vi "Joystick_Operation.vi"(0 "System no.":i32=1 min=1 step=1, 1 "Joystick ID":u32, 2 "X axis":string="B", 3 "Y axis":string="E", 4 "No.of digits for MOV command":i16=2, 5 "error in":errorcluster, 6 "Resolution factor X":i32=150, 7 "Resolution factor Y":i32=150, 8 "Dead band X":i32=2, 9 "Dead band Y":i32=2, 10 "Use #24 for Stop?":bool=TRUE, 11 "Read from controller?":bool=TRUE caption="Read travel range\nfrom controller?", 12 "Maximum velocity values":T2={"Velocity1 X"=1.0, "Velocity2 X"=20.0, "Velocity1 Y"=0.5, "Velocity2 Y"=15.0} {"Velocity2 Y" format="%.6f"; "Velocity1 Y" format="%.6f"; "Velocity2 X" format="%.6f"; "Velocity1 X" format="%.6f"}, 13 "Travel range":T1={"Xmax"=10.0, "Xmin"=0.0, "Ymax"=5.0, "Ymin"=0.0} {"Ymin" format="%.6f"; "Ymax" format="%.6f"; "Xmin" format="%.6f"; "Xmax" format="%.6f"}, 14 "System no. 2":i32=1 min=1 step=1) -> (19 "error out":errorcluster)   [LabVIEW 2020]
doc: "This VI can be used to control two closed-loop axes (which can belong to one or two connected systems) with a 2-button, 2-axis joystick connected to the host computer. The absolute value of the joystick position is converted into velocity values for the two stages connected to the system being commanded. Two velocity levels for each axis can be specified, e.g. one for fast, rough positioning and one for slow, fine positioning. Joystick button 2 switches between these levels. The sign of the joystick position determines whether the move command issued contains the positive or negative travel limit (read automatically if Read travel range from controller? is TRUE) of the corresponding axis. When the joystick is \"in the middle position\", the velocity of the corresponding axis is set to zero. \nDead band * is the maximum size of the scaled joystick position value that does not result in any motion. \nResolution factor * determines the joystick resolution. \nNo. of digits is the number of digits after the decimal point in the position values that will be sent by the MOV command. \nIf joystick button 1 is pressed, a stop command (STP or #24, depending on Use 24 for stop) is sent to the controller. The diagram shows how to combine the driver and support VIs for these tasks. \n\nIf only one motion axis is to be controlled, Y Axis must be identical to X Axis, System no. 2 must be identical to System no. 1, and Y axis of joystick is to be used for control of the motion axis.\n\nIf required: Install the joystick driver and calibrate the joystick in the Windows control panel before running this VI.\n\nRun PI_GCS2_Configuration_setup.vi prior to running this VI."
uses:
  Low Level/General command.llb/Controller names.ctl
  Low Level/General command.llb/Global2 (Array).vi
panel:
  out "Current Vy":dbl(slide) scale=0.0..0.5 scale format="%.4f"
  out "Current Vx":dbl(slide) scale=0.0..1.0 scale format="%.4f"
  out "Position plot":cluster{dbl[], dbl[]}(graph)
  out "Current pos. Y":dbl format="%.2f"
  out "Current pos. X":dbl format="%.2f"
  out "Current Vy":dbl format="%.6f"
  out "Current Vx":dbl format="%.6f"
  out "Current Vy, max":dbl format="%.6f"
  out "Current Vx, max":dbl format="%.6f"
  in  "stop":bool
  out "JoyY":i32
  out "JoyX":i32
  out "JoyY scaled":i32
  out "JoyX scaled":i32
  # "Joystick operation sample program."
  # "Install joystick driver, calibrate joystick in the Windows control \tpanel and run \"Configuration_Setup.vi\" before running this VI. Use joystick button 1\nto stop motion of both axes and button2 to switch between two velocity levels. If only one motion axis is to be controlled, Y Axis must be identical\nto X Axis, System no. 2 must be identical to System no. 1, and Y axis of joystick is to be used for control of the motion axis.See VI and control/\nindicator information for details."
  # "For X axis:"
  # "For Y axis:"
  # "Joystick axes settings"
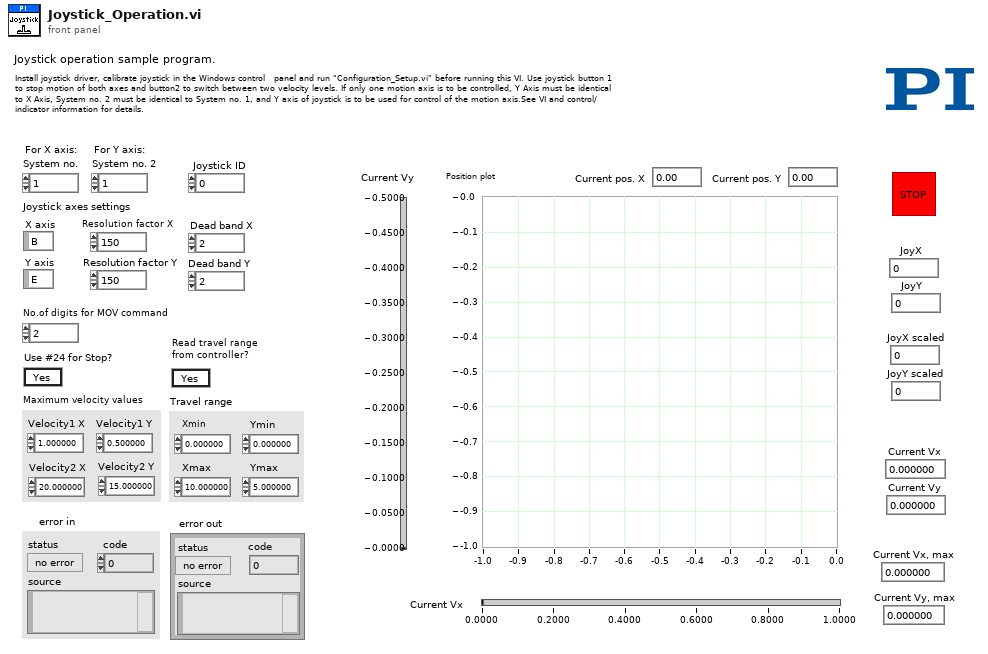
[diagram p1: front panel]
types:
  T1 = cluster{"Xmax":dbl, "Xmin":dbl, "Ymax":dbl, "Ymin":dbl}
  T2 = cluster{"Velocity1 X":dbl, "Velocity2 X":dbl, "Velocity1 Y":dbl, "Velocity2 Y":dbl}
  T3 = typedef "Controller names.ctl" = enum16{"None", "Analog", "C-702", "C-413", "C-414", "C-843", "C-843.PM", "C-844", "C-848", "C-865", "C-866", "C-867", "C-877", "C-880", "C-884", "C-885", "C-886", "C-887", "C-891", "E-135", "E-516", "E-517", "E-518", "E-709", "E-710", "E-712", "E-725", "E-727", "E-753", "E-754", "E-755", "E-761", "E-816", "E-861", "E-870", "E-871", "E-872", "E-873", "E-874", "F-206", "HydraPollux", "M-840", "M-850", "M-8X0", "Mercury", "Mercury_GCS", "PI_GCS2"}
  T4 = cluster{"Conn. axes":string[], "Controller name":T3}[]
  T5 = cluster{"Conn. axes":string[], "Controller name":T3}
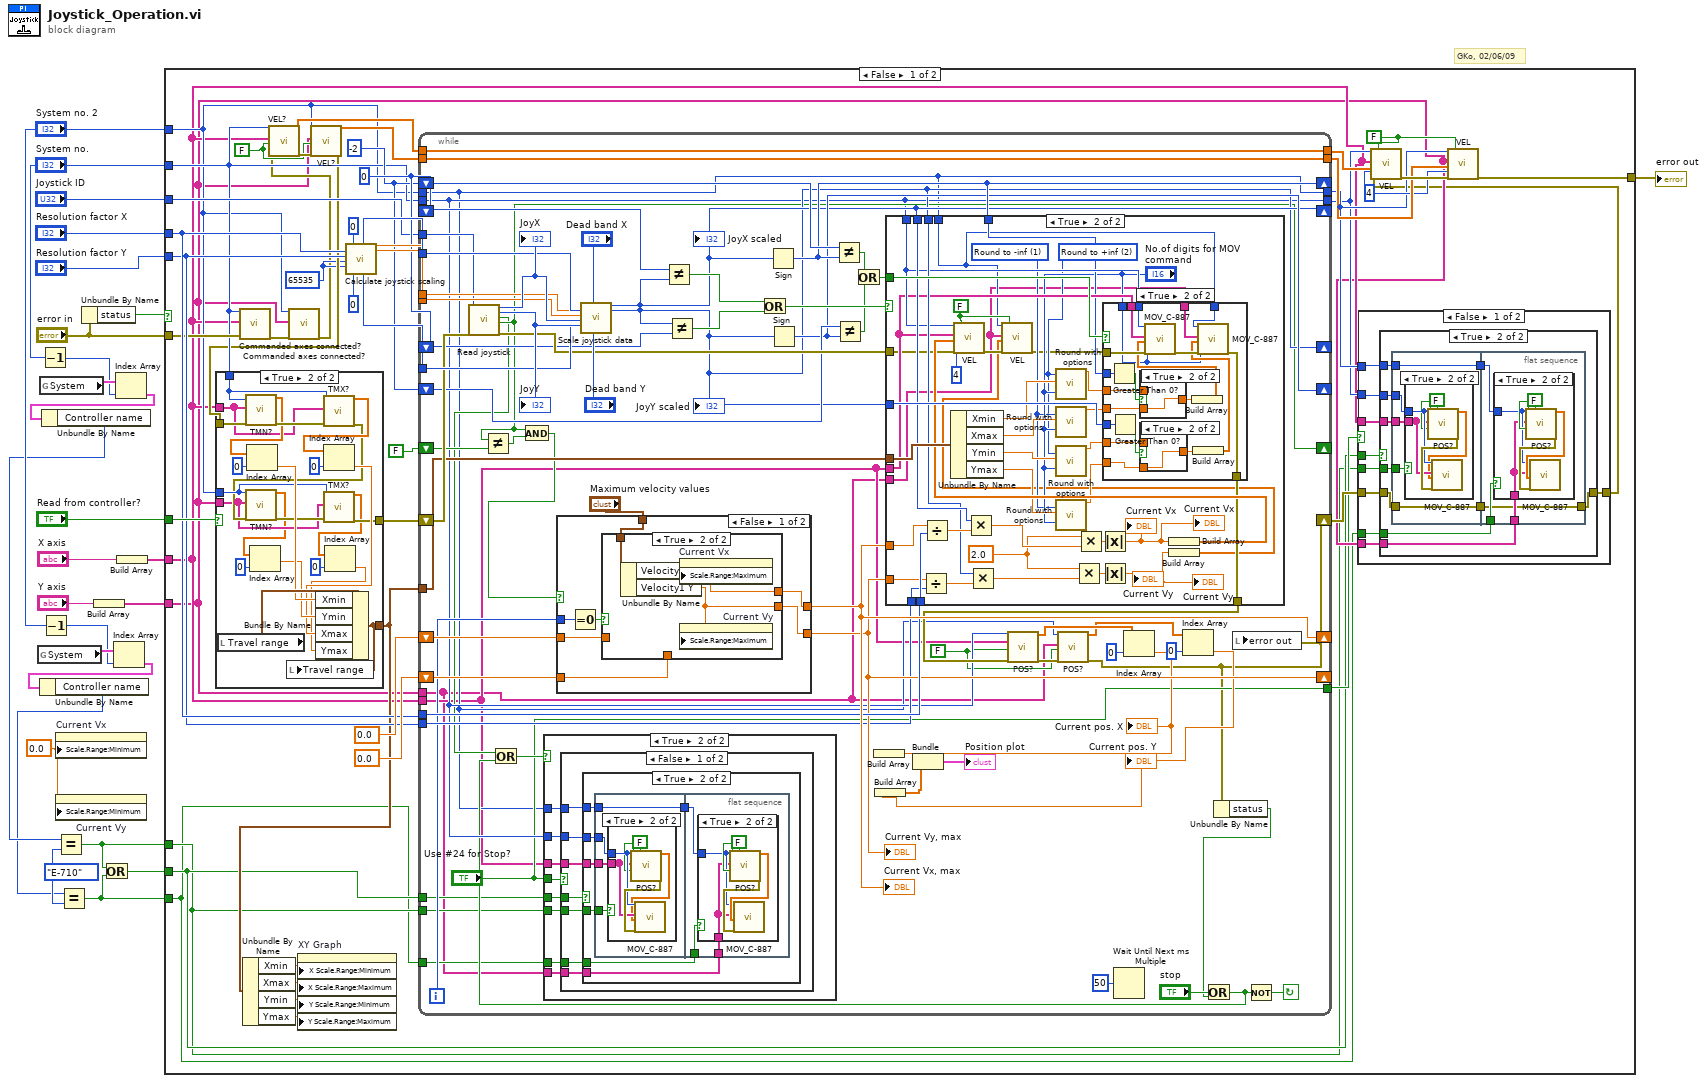
[diagram p0: block diagram]
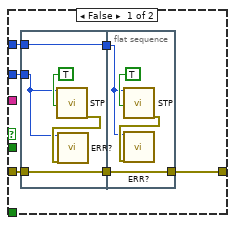
[diagram p2: hidden frame]
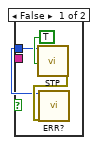
[diagram p3: hidden frame]
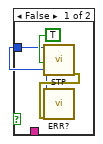
[diagram p4: hidden frame]
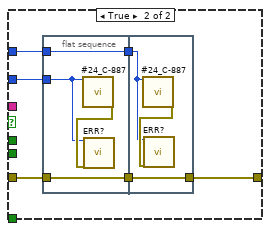
[diagram p5: hidden frame]
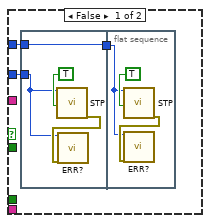
[diagram p11: hidden frame]
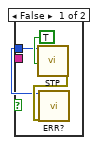
[diagram p12: hidden frame]
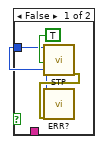
[diagram p13: hidden frame]
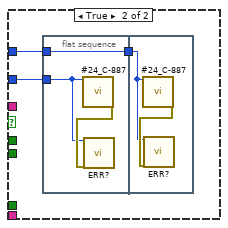
[diagram p14: hidden frame]
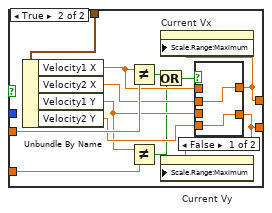
[diagram p16: hidden frame]
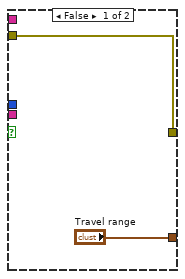
[diagram p18: hidden frame]
diagram:
  w6 = Controller_names."E-710" ("Controller name")
  w19 = 0.0 ("Write Attribute")
  # "GKo, 02/06/09"
  n1 = global read "Global2 (Array).vi" "System"() -> (w9:T4)
  n2 = Decrement(x="System no.") -> (x-1=w11:i32)
  n3 = global read "Global2 (Array).vi" "System"() -> (w14:T4)
  n4 = Decrement(x="System no. 2") -> (x-1=w8:i32)
  n5 = property on="Current Vx" class="Slide (strict)"("Scale.Range:Minimum"=w19) -> ()  [unwired: 2 in, 2 out]
  n6 = property on="Current Vy" class="Slide (strict)"("Scale.Range:Minimum"=w19) -> ()  [unwired: 2 in, 2 out]
  n7 = Unbundle By Name("error in") -> ("status"=w21:bool)
  n8 = Build Array("Y axis") -> (w15:string[])
  n9 = Index Array(array=w9, index=w8) -> (element=w7:T5)
  n10 = Unbundle By Name(w7) -> ("Controller name"=w4:T3)
  n11 = Equal?(x=w4, y=w6) -> (x = y?=w2:bool)
  n12 = Index Array(array=w14, index=w11) -> (element=w10:T5)
  n13 = Unbundle By Name(w10) -> ("Controller name"=w5:T3)
  n14 = Equal?(x=w5, y=w6) -> (x = y?=w3:bool)
  n15 = Or(x=w3, y=w2) -> (x .or. y?=w1:bool)
  n16 = Build Array("X axis") -> (w16:string[])
  n17 = case shown="False" w21 {
    tunnel: "Resolution factor X" -> [w61 _]
    tunnel: "Resolution factor Y" -> [w60 _]
    tunnel: "System no." -> [w52 _]
    tunnel: [w39 w399] -> w24
    tunnel: "Read from controller?" -> [w65 _]
    tunnel: "error in" -> [w59 w399]
    tunnel: "Joystick ID" -> [w63 _]
    tunnel: w16 -> [w33 _]
    tunnel: w15 -> [w32 _]
    tunnel: "System no. 2" -> [w41 _]
    tunnel: w2 -> [w28 _]
    tunnel: w3 -> [w29 _]
    tunnel: w1 -> [w30 _]
    frame False {
      w37 = i16 4 ("No.of digits")
      w62 = -2
      w64 = 0 ("XPos scaled")
      w44 = FALSE ("All axes?")
      w49 = FALSE ("Without axis ID?")
      w45 = 65535 ("XPos max")
      n18 = call "Commanded axes connected?.vi"("System no."=w52, "Commanded axes"=w33, "error in"=w59) -> ("error out"=w43:errorcluster)  [unwired: 16 out]
      n19 = call "Commanded axes connected?.vi"("System no."=w41, "Commanded axes"=w32, "error in"=w43) -> ("error out"=w42:errorcluster)  [unwired: 16 out]
      n20 = call "VEL?.vi"("System no."=w52, "Axes to query"=w33, "All axes?"=w44, "error in"=w42) -> ("Velocity"=w51:dbl[], "error out"=w47:errorcluster)  [unwired: 1 in, 13 out]
      n21 = call "VEL?.vi"("System no."=w41, "Axes to query"=w32, "All axes?"=w44, "error in"=w47) -> ("Velocity"=w48:dbl[], "error out"=w46:errorcluster)  [unwired: 1 in, 13 out]
      n22 = case shown="True" w65 {
        tunnel: ["Travel range" w385] -> w58
        tunnel: w46 -> [w374 w397]
        tunnel: [w374 w379] -> w66
        tunnel: w52 -> [_ w396]
        tunnel: w33 -> [_ w384]
        tunnel: w41 -> [_ w382]
        tunnel: w32 -> [_ w378]
        frame False {
        }
        frame True {
          n23 = local read "Travel range"() -> (w391:T1)
          n24 = call "TMN?.vi"("System no."=w396, "Axes to query"=w384, "error in"=w397) -> ("Minimum travel limit"=w395:dbl[], "error out"=w398:errorcluster)  [unwired: 2 in, 13 out]
          n25 = Index Array(array=w395, index=0 ("Index")) -> (element=w390:dbl)
          n26 = call "TMX?.vi"("System no."=w396, "Axes to query"=w384, "error in"=w398) -> ("Maximum travel limit"=w389:dbl[], "error out"=w381:errorcluster)  [unwired: 2 in, 13 out]
          n27 = call "TMN?.vi"("System no."=w382, "Axes to query"=w378, "error in"=w381) -> ("Minimum travel limit"=w377:dbl[], "error out"=w380:errorcluster)  [unwired: 2 in, 13 out]
          n28 = Index Array(array=w377, index=0 ("Index")) -> (element=w388:dbl)
          n29 = Index Array(array=w389, index=0 ("Index")) -> (element=w387:dbl)
          n30 = call "TMX?.vi"("System no."=w382, "Axes to query"=w378, "error in"=w380) -> ("Maximum travel limit"=w376:dbl[], "error out"=w379:errorcluster)  [unwired: 2 in, 13 out]
          n31 = Index Array(array=w376, index=0 ("Index")) -> (element=w386:dbl)
          n32 = Bundle By Name(cluster=w391, "Xmin"=w390, "Ymin"=w388, "Xmax"=w387, "Ymax"=w386) -> (w385:T1)
          n33 = local write "Travel range"(w385) -> ()
        }
      }
      n34 = Unbundle By Name(w58) -> ("Xmin"=w57:dbl, "Xmax"=w56:dbl, "Ymin"=w55:dbl, "Ymax"=w54:dbl)
      n35 = property on="XY Graph" class="XYGraph (strict)"("X Scale.Range:Minimum"=w57, "X Scale.Range:Maximum"=w56, "Y Scale.Range:Minimum"=w55, "Y Scale.Range:Maximum"=w54) -> ()  [unwired: 2 in, 2 out]
      n36 = call "Calculate joystick scaling.vi"("Resolution factor X"=w61, "Resolution factor Y"=w60, "XPos max"=w45, "YPos max"=w45, "XPos min"=0, "YPos min"=0) -> ("XPos Center scaled"=w72:i32, "YPos Center scaled"=w71:i32, "Scaling factor X"=w70:dbl, "Scaling factor Y"=w69:dbl)  [unwired: 10 out]
      n37 = while {
        tunnel: ["Use #24 for Stop?"] -> w31
        tunnel: [w162] -> w50
        tunnel: [w163] -> w34
        tunnel: w51 -> [w162]
        shift-left: FALSE ("Button 2 pressed") -> [w167]
        shift-right: [w165] -> _
        tunnel: w60 -> [w180]
        tunnel: w61 -> [w182]
        shift-left: w62 -> [w188]
        shift-right: [w184] -> _
        shift-left: w62 -> [w189]
        shift-right: [w186] -> _
        tunnel: w63 -> [w193]
        shift-left: w64 -> [w197]
        shift-right: [w179] -> _
        shift-left: w64 -> [w196]
        shift-right: [w178] -> _
        tunnel: w33 -> [w149]
        tunnel: w58 -> [w185]
        shift-left: 0.0 -> [w202]
        shift-right: [w181] -> _
        shift-left: 0.0 -> [w203]
        shift-right: [w183] -> _
        shift-left: w66 -> [w198]
        shift-right: [w155] -> w36
        tunnel: w52 -> [w163]
        tunnel: w69 -> [w207]
        tunnel: w70 -> [w210]
        tunnel: w71 -> [w211]
        tunnel: w72 -> [w212]
        tunnel: w48 -> [w157]
        tunnel: w41 -> [w152]
        tunnel: [w152] -> w35
        tunnel: [w157] -> w38
        tunnel: w32 -> [w147]
        tunnel: w30 -> [w151]
        tunnel: w29 -> [w150]
        tunnel: w28 -> [w148]
        i -> [w177]
        stop <- w206 continue-if-true
        w154 = FALSE ("All axes?")
        n38 = call "Read joystick.vi"("Joystick ID"=w193, "error in"=w198) -> ("XPos"=w214:i32, "YPos"=w213:i32, "Button 1 pressed"=w161:bool, "Button 2 pressed"=w165:bool, "error out"=w199:errorcluster)  [unwired: 13 out]
        "JoyX" <- w214
        "JoyY" <- w213
        n39 = Not Equal?(x=w165, y=w167) -> (x != y?=w166:bool)
        n40 = And(x=w165, y=w166) -> (x .and. y?=w164:bool)
        n41 = case shown="False" w164 {
          tunnel: "Maximum velocity values" -> [w350 w369]
          tunnel: w203 -> [w348 w368]
          tunnel: [w349 w359] -> w183
          tunnel: w202 -> [w346 w363]
          tunnel: [w347 w358] -> w181
          tunnel: w177 -> [w352 _]
          frame False {
            n42 = Equal To 0?(x=w352) -> (x = 0?=w351:bool)
            n43 = case shown="True" w351 {
              tunnel: w350 -> [_ w357]
              tunnel: [w354 w355] -> w349
              tunnel: w348 -> [w354 _]
              tunnel: [w353 w356] -> w347
              tunnel: w346 -> [w353 _]
              frame False {
              }
              frame True {
                n44 = Unbundle By Name(w357) -> ("Velocity1 X"=w355:dbl, "Velocity1 Y"=w356:dbl)
                n45 = property on="Current Vx" class="Slide (strict)"("Scale.Range:Maximum"=w355) -> ()  [unwired: 2 in, 2 out]
                n46 = property on="Current Vy" class="Slide (strict)"("Scale.Range:Maximum"=w356) -> ()  [unwired: 2 in, 2 out]
              }
            }
          }
          frame True {
            n47 = Unbundle By Name(w369) -> ("Velocity1 X"=w367:dbl, "Velocity2 X"=w366:dbl, "Velocity1 Y"=w364:dbl, "Velocity2 Y"=w365:dbl)
            n48 = Not Equal?(x=w367, y=w368) -> (x != y?=w362:bool)
            n49 = Not Equal?(x=w364, y=w363) -> (x != y?=w361:bool)
            n50 = Or(x=w362, y=w361) -> (x .or. y?=w360:bool)
            n51 = case shown="False" w360 {
              tunnel: [w371 w373] -> w359
              tunnel: w367 -> [_ w373]
              tunnel: w366 -> [w371 _]
              tunnel: w365 -> [w370 _]
              tunnel: [w370 w372] -> w358
              tunnel: w364 -> [_ w372]
              frame False {
              }
              frame True {
              }
            }
            n52 = property on="Current Vx" class="Slide (strict)"("Scale.Range:Maximum"=w359) -> ()  [unwired: 2 in, 2 out]
            n53 = property on="Current Vy" class="Slide (strict)"("Scale.Range:Maximum"=w358) -> ()  [unwired: 2 in, 2 out]
          }
        }
        "Current Vx, max" <- w183
        "Current Vy, max" <- w181
        n54 = call "Scale joystick data.vi"("Factor X"=w210, "Factor Y"=w207, "XPos"=w214, "YPos"=w213, "XPos Center"=w212, "YPos Center"=w211, "Dead band X"="Dead band X", "Dead band Y"="Dead band Y") -> ("XPos scaled"=w179:i32, "YPos scaled"=w178:i32)  [unwired: 10 out]
        "JoyX scaled" <- w179
        "JoyY scaled" <- w178
        n55 = Not Equal?(x=w197, y=w179) -> (x != y?=w195:bool)
        n56 = Not Equal?(x=w178, y=w196) -> (x != y?=w194:bool)
        n57 = Or(x=w195, y=w194) -> (x .or. y?=w192:bool)
        n58 = Sign(1:w179) -> (0:w186:i32)
        n59 = Sign(1:w178) -> (0:w184:i32)
        n60 = Not Equal?(x=w189, y=w186) -> (x != y?=w191:bool)
        n61 = Not Equal?(x=w188, y=w184) -> (x != y?=w190:bool)
        n62 = Or(x=w191, y=w190) -> (x .or. y?=w187:bool)
        n63 = case shown="True" w192 {
          tunnel: [w215 w237] -> w174
          tunnel: w199 -> [w215 w235]
          tunnel: w163 -> [_ w239]
          tunnel: w149 -> [_ w238]
          tunnel: w187 -> [_ w256]
          tunnel: w186 -> [_ w234]
          tunnel: w178 -> [_ w255]
          tunnel: w185 -> [_ w254]
          tunnel: w183 -> [_ w253]
          tunnel: w182 -> [_ w252]
          tunnel: w181 -> [_ w251]
          tunnel: w180 -> [_ w250]
          tunnel: w179 -> [_ w247]
          tunnel: w178 -> [_ w246]
          tunnel: w152 -> [_ w217]
          tunnel: w147 -> [_ w216]
          frame False {
          }
          frame True {
            w223 = u16 2 items=["Round to nearest", "Round to -inf", "Round to +inf"] ("Round mode selection")
            w224 = u16 1 items=["Round to nearest", "Round to -inf", "Round to +inf"] ("Round mode selection")
            w240 = 2.0 ("x")
            w220 = FALSE ("Without axis ID?")
            n64 = Divide(x=w251, y=w250) -> (x/y=w248:dbl)
            n65 = Divide(x=w253, y=w252) -> (x/y=w249:dbl)
            n66 = Unbundle By Name(w254) -> ("Xmin"=w233:dbl, "Xmax"=w231:dbl, "Ymin"=w229:dbl, "Ymax"=w227:dbl)
            n67 = Multiply(x=w247, y=w249) -> (x*y=w245:dbl)
            n68 = Multiply(x=w246, y=w248) -> (x*y=w244:dbl)
            n69 = call "Round with options.vi"("Round mode selection"=w223, "Numeric in"=w233, "No.of digits\nto round to"="No.of digits for MOV command") -> ("Numeric out"=w232:dbl)  [unwired: 1 in, 15 out]
            n70 = call "Round with options.vi"("Round mode selection"=w224, "Numeric in"=w231, "No.of digits\nto round to"="No.of digits for MOV command") -> ("Numeric out"=w230:dbl)  [unwired: 1 in, 15 out]
            n71 = call "Round with options.vi"("Round mode selection"=w223, "Numeric in"=w229, "No.of digits\nto round to"="No.of digits for MOV command") -> ("Numeric out"=w228:dbl)  [unwired: 1 in, 15 out]
            n72 = call "Round with options.vi"("Round mode selection"=w224, "Numeric in"=w227, "No.of digits\nto round to"="No.of digits for MOV command") -> ("Numeric out"=w226:dbl)  [unwired: 1 in, 15 out]
            n73 = Multiply(x=w240, y=w244) -> (x*y=w241:dbl)
            n74 = Multiply(x=w240, y=w245) -> (x*y=w242:dbl)
            n75 = Absolute Value(x=w242) -> (abs(x)=w236:dbl)
            "Current Vx" <- w236
            "Current Vx" <- w236
            n76 = Absolute Value(x=w241) -> (abs(x)=w219:dbl)
            "Current Vy" <- w219
            "Current Vy" <- w219
            n77 = Build Array(w236) -> (w243:dbl[])
            n78 = call "VEL.vi"("System no."=w239, "Axes to set"=w238, "Velocity values"=w243, "No.of digits"=i16 4, "error in"=w235, "Without axis ID?"=w220) -> ("error out"=w222:errorcluster)  [unwired: 13 out]
            n79 = Build Array(w219) -> (w218:dbl[])
            n80 = call "VEL.vi"("System no."=w217, "Axes to set"=w216, "Velocity values"=w218, "error in"=w222, "Without axis ID?"=w220) -> ("error out"=w221:errorcluster)  [unwired: 1 in, 13 out]
            n81 = case shown="True" w256 {
              tunnel: [w258 w263] -> w237
              tunnel: "No.of digits for MOV command" -> [_ w259]
              tunnel: w221 -> [w258 w278]
              tunnel: w239 -> [_ w277]
              tunnel: w238 -> [_ w276]
              tunnel: w234 -> [_ w275]
              tunnel: w255 -> [_ w274]
              tunnel: w230 -> [_ w272]
              tunnel: w232 -> [_ w271]
              tunnel: w228 -> [_ w269]
              tunnel: w226 -> [_ w268]
              tunnel: w217 -> [_ w262]
              tunnel: w216 -> [_ w261]
              frame False {
              }
              frame True {
                n82 = Greater Than 0?(x=w275) -> (x > 0?=w273:bool)
                n83 = Greater Than 0?(x=w274) -> (x > 0?=w270:bool)
                n84 = case shown="True" w273 {
                  tunnel: w272 -> [_ w282]
                  tunnel: w271 -> [w281 _]
                  tunnel: [w281 w282] -> w267
                  frame False {
                  }
                  frame True {
                  }
                }
                n85 = case shown="True" w270 {
                  tunnel: w269 -> [w279 _]
                  tunnel: w268 -> [_ w280]
                  tunnel: [w279 w280] -> w265
                  frame False {
                  }
                  frame True {
                  }
                }
                n86 = Build Array(w267) -> (w266:dbl[])
                n87 = call "MOV_C-887.vi"("System no."=w277, "Axes to move"=w276, "Position values"=w266, "No.of digits"=w259, "error in"=w278) -> ("error out"=w264:errorcluster)  [unwired: 14 out]
                n88 = Build Array(w265) -> (w260:dbl[])
                n89 = call "MOV_C-887.vi"("System no."=w262, "Axes to move"=w261, "Position values"=w260, "No.of digits"=w259, "error in"=w264) -> ("error out"=w263:errorcluster)  [unwired: 14 out]
              }
            }
          }
        }
        n90 = call "POS?.vi"("System no."=w163, "Axes to query"=w149, "All axes?"=w154, "error in"=w174) -> ("Position"=w173:dbl[], "error out"=w156:errorcluster)  [unwired: 1 in, 13 out]
        n91 = call "POS?.vi"("System no."=w152, "Axes to query"=w147, "All axes?"=w154, "error in"=w156) -> ("Position"=w153:dbl[], "error out"=w155:errorcluster)  [unwired: 1 in, 13 out]
        n92 = Wait Until Next ms Multiple(millisecond multiple=u32 50) -> ()  [unwired: 1 out]
        n93 = Index Array(array=w173, index=0 ("Index")) -> (element=w172:dbl)
        "Current pos. X" <- w172
        n94 = Build Array(w172) -> (w170:dbl[])
        n95 = Index Array(array=w153, index=0 ("Index")) -> (element=w171:dbl)
        "Current pos. Y" <- w171
        n96 = Build Array(w171) -> (w169:dbl[])
        n97 = Bundle(w170, w169) -> (→"Position plot":cluster{dbl[], dbl[]})  [unwired: 1 out]
        n98 = Unbundle By Name(w155) -> ("status"=w200:bool)
        n99 = Or(x="stop", y=w200) -> (x .or. y?=w160:bool)
        n100 = Or(x=w161, y=w160) -> (x .or. y?=w159:bool)
        n101 = case shown="True" w159 {
          tunnel: w163 -> [_ w290]
          tunnel: "Use #24 for Stop?" -> [_ w289]
          tunnel: w152 -> [_ w288]
          tunnel: w151 -> [_ w287]
          tunnel: w150 -> [_ w286]
          tunnel: w149 -> [_ w285]
          tunnel: w148 -> [_ w284]
          tunnel: w147 -> [_ w283]
          frame False {
          }
          frame True {
            n102 = case shown="False" w289 {
              tunnel: w290 -> [w297 w338]
              tunnel: w288 -> [w296 w339]
              tunnel: w287 -> [w295 _]
              tunnel: w286 -> [w294 _]
              tunnel: w285 -> [w293 _]
              tunnel: w284 -> [w292 _]
              tunnel: w283 -> [w291 _]
              frame False {
                n103 = case shown="True" w295 {
                  tunnel: w297 -> [w299 w313]
                  tunnel: w296 -> [w298 w312]
                  tunnel: w294 -> [_ w311]
                  tunnel: w293 -> [_ w310]
                  tunnel: w292 -> [_ w309]
                  tunnel: w291 -> [_ w308]
                  frame False {
                    n104 = flat-sequence {
                      tunnel: w298 -> [w301]
                      tunnel: [w301] -> w300
                      tunnel: w299 -> [w302]
                      tunnel: w300 -> [w305]
                      frame #0 {
                        n105 = call "STP.vi"("System no."=w302, "All axes?"=TRUE) -> ("error out"=w304:errorcluster)  [unwired: 1 in, 16 out]
                        n106 = call "ERR?.vi"("System no."=w302, "error in"=w304) -> ()  [unwired: 18 out]
                      }
                      frame #1 {
                        n107 = call "STP.vi"("System no."=w305, "All axes?"=TRUE) -> ("error out"=w306:errorcluster)  [unwired: 1 in, 16 out]
                        n108 = call "ERR?.vi"("System no."=w305, "error in"=w306) -> ()  [unwired: 18 out]
                      }
                    }
                  }
                  frame True {
                    n109 = flat-sequence {
                      tunnel: w312 -> [w317]
                      tunnel: [w317] -> w314
                      tunnel: w313 -> [w318]
                      tunnel: w311 -> [w316]
                      tunnel: w310 -> [w315]
                      tunnel: w314 -> [w329]
                      tunnel: w309 -> [w328]
                      tunnel: w308 -> [w327]
                      frame #0 {
                        n110 = case shown="True" w316 {
                          tunnel: w318 -> [w319 w325]
                          tunnel: w315 -> [_ w323]
                          frame False {
                            n111 = call "STP.vi"("System no."=w319, "All axes?"=TRUE) -> ("error out"=w321:errorcluster)  [unwired: 1 in, 16 out]
                            n112 = call "ERR?.vi"("System no."=w319, "error in"=w321) -> ()  [unwired: 18 out]
                          }
                          frame True {
                            n113 = call "POS?.vi"("System no."=w325, "Axes to query"=w323, "All axes?"=FALSE) -> ("Position"=w322:dbl[], "error out"=w326:errorcluster)  [unwired: 2 in, 13 out]
                            n114 = call "MOV_C-887.vi"("System no."=w325, "Axes to move"=w323, "Position values"=w322, "error in"=w326) -> ()  [unwired: 1 in, 15 out]
                          }
                        }
                      }
                      frame #1 {
                        n115 = case shown="True" w328 {
                          tunnel: w329 -> [w330 w334]
                          tunnel: w327 -> [_ w333]
                          frame False {
                            n116 = call "STP.vi"("System no."=w330, "All axes?"=TRUE) -> ("error out"=w331:errorcluster)  [unwired: 1 in, 16 out]
                            n117 = call "ERR?.vi"("System no."=w330, "error in"=w331) -> ()  [unwired: 18 out]
                          }
                          frame True {
                            n118 = call "POS?.vi"("System no."=w334, "Axes to query"=w333, "All axes?"=FALSE) -> ("Position"=w337:dbl[], "error out"=w335:errorcluster)  [unwired: 2 in, 13 out]
                            n119 = call "MOV_C-887.vi"("System no."=w334, "Axes to move"=w333, "Position values"=w337, "error in"=w335) -> ()  [unwired: 1 in, 15 out]
                          }
                        }
                      }
                    }
                  }
                }
              }
              frame True {
                n120 = flat-sequence {
                  tunnel: w339 -> [w342]
                  tunnel: [w342] -> w340
                  tunnel: w338 -> [w341]
                  tunnel: w340 -> [w344]
                  frame #0 {
                    n121 = call "#24_C-887.vi"("System no."=w341) -> ("error out"=w343:errorcluster)  [unwired: 1 in, 17 out]
                    n122 = call "ERR?.vi"("System no."=w341, "error in"=w343) -> ()  [unwired: 18 out]
                  }
                  frame #1 {
                    n123 = call "#24_C-887.vi"("System no."=w344) -> ("error out"=w345:errorcluster)  [unwired: 1 in, 17 out]
                    n124 = call "ERR?.vi"("System no."=w344, "error in"=w345) -> ()  [unwired: 18 out]
                  }
                }
              }
            }
          }
        }
        n125 = local write "error out"(w155) -> ()
        n126 = Not(x=w160) -> (.not. x?=w206:bool)
      }
      n127 = case shown="False" w31 {
        tunnel: w34 -> [w83 w137]
        tunnel: w35 -> [w82 w138]
        tunnel: w30 -> [w81 _]
        tunnel: w29 -> [w80 _]
        tunnel: w33 -> [w79 _]
        tunnel: w28 -> [w78 _]
        tunnel: w32 -> [w77 _]
        tunnel: [w76 w136] -> w27
        tunnel: w36 -> [w75 w134]
        frame False {
          n128 = case shown="True" w81 {
            tunnel: w83 -> [w88 w107]
            tunnel: w82 -> [w87 w106]
            tunnel: w80 -> [_ w105]
            tunnel: w79 -> [_ w104]
            tunnel: w78 -> [_ w103]
            tunnel: w77 -> [_ w102]
            tunnel: [w86 w101] -> w76
            tunnel: w75 -> [w84 w99]
            frame False {
              n129 = flat-sequence {
                tunnel: w87 -> [w91]
                tunnel: [w91] -> w89
                tunnel: w88 -> [w92]
                tunnel: w84 -> [w90]
                tunnel: [w90] -> w85
                tunnel: w89 -> [w96]
                tunnel: [w95] -> w86
                tunnel: w85 -> [w95]
                frame #0 {
                  n130 = call "STP.vi"("System no."=w92, "All axes?"=TRUE) -> ("error out"=w94:errorcluster)  [unwired: 1 in, 16 out]
                  n131 = call "ERR?.vi"("System no."=w92, "error in"=w94) -> ()  [unwired: 18 out]
                }
                frame #1 {
                  n132 = call "STP.vi"("System no."=w96, "All axes?"=TRUE) -> ("error out"=w97:errorcluster)  [unwired: 1 in, 16 out]
                  n133 = call "ERR?.vi"("System no."=w96, "error in"=w97) -> ()  [unwired: 18 out]
                }
              }
            }
            frame True {
              n134 = flat-sequence {
                tunnel: w106 -> [w112]
                tunnel: [w112] -> w108
                tunnel: w107 -> [w113]
                tunnel: w105 -> [w111]
                tunnel: w104 -> [w110]
                tunnel: w99 -> [w109]
                tunnel: [w109] -> w100
                tunnel: w108 -> [w125]
                tunnel: w103 -> [w124]
                tunnel: w102 -> [w123]
                tunnel: [w122] -> w101
                tunnel: w100 -> [w122]
                frame #0 {
                  n135 = case shown="True" w111 {
                    tunnel: w113 -> [w114 w120]
                    tunnel: w110 -> [_ w118]
                    frame False {
                      n136 = call "STP.vi"("System no."=w114, "All axes?"=TRUE) -> ("error out"=w116:errorcluster)  [unwired: 1 in, 16 out]
                      n137 = call "ERR?.vi"("System no."=w114, "error in"=w116) -> ()  [unwired: 18 out]
                    }
                    frame True {
                      n138 = call "POS?.vi"("System no."=w120, "Axes to query"=w118, "All axes?"=FALSE) -> ("Position"=w117:dbl[], "error out"=w121:errorcluster)  [unwired: 2 in, 13 out]
                      n139 = call "MOV_C-887.vi"("System no."=w120, "Axes to move"=w118, "Position values"=w117, "error in"=w121) -> ()  [unwired: 1 in, 15 out]
                    }
                  }
                }
                frame #1 {
                  n140 = case shown="True" w124 {
                    tunnel: w125 -> [w126 w130]
                    tunnel: w123 -> [_ w129]
                    frame False {
                      n141 = call "STP.vi"("System no."=w126, "All axes?"=TRUE) -> ("error out"=w127:errorcluster)  [unwired: 1 in, 16 out]
                      n142 = call "ERR?.vi"("System no."=w126, "error in"=w127) -> ()  [unwired: 18 out]
                    }
                    frame True {
                      n143 = call "POS?.vi"("System no."=w130, "Axes to query"=w129, "All axes?"=FALSE) -> ("Position"=w133:dbl[], "error out"=w131:errorcluster)  [unwired: 2 in, 13 out]
                      n144 = call "MOV_C-887.vi"("System no."=w130, "Axes to move"=w129, "Position values"=w133, "error in"=w131) -> ()  [unwired: 1 in, 15 out]
                    }
                  }
                }
              }
            }
          }
        }
        frame True {
          n145 = flat-sequence {
            tunnel: w138 -> [w142]
            tunnel: [w142] -> w139
            tunnel: w137 -> [w141]
            tunnel: w134 -> [w140]
            tunnel: [w140] -> w135
            tunnel: w139 -> [w145]
            tunnel: [w144] -> w136
            tunnel: w135 -> [w144]
            frame #0 {
              n146 = call "#24_C-887.vi"("System no."=w141) -> ("error out"=w143:errorcluster)  [unwired: 1 in, 17 out]
              n147 = call "ERR?.vi"("System no."=w141, "error in"=w143) -> ()  [unwired: 18 out]
            }
            frame #1 {
              n148 = call "#24_C-887.vi"("System no."=w145) -> ("error out"=w146:errorcluster)  [unwired: 1 in, 17 out]
              n149 = call "ERR?.vi"("System no."=w145, "error in"=w146) -> ()  [unwired: 18 out]
            }
          }
        }
      }
      n150 = call "VEL.vi"("System no."=w34, "Axes to set"=w33, "Velocity values"=w50, "No.of digits"=w37, "error in"=w27, "Without axis ID?"=w49) -> ("error out"=w40:errorcluster)  [unwired: 13 out]
      n151 = call "VEL.vi"("System no."=w35, "Axes to set"=w32, "Velocity values"=w38, "No.of digits"=w37, "error in"=w40, "Without axis ID?"=w49) -> ("error out"=w39:errorcluster)  [unwired: 13 out]
    }
    frame True {
    }
  }
  "error out" <- w24
